vi "process.vi"(1 "input":dbl[][](array[numeric])) -> (0 "xxxx":dbl[][](array[numeric]))   [LabVIEW 2022 SP3]
uses:
  <vilib>/Analysis/NI_AALBase.lvlib
panel:
  out "mean&std":dbl[][](array[numeric])
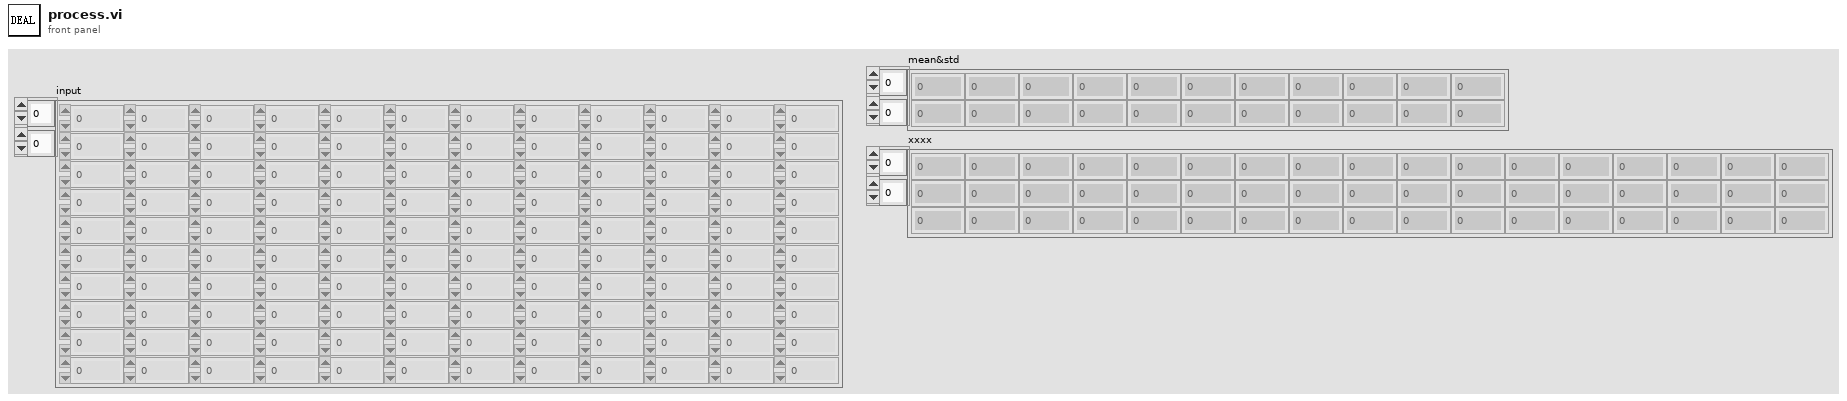
[diagram p1: front panel]
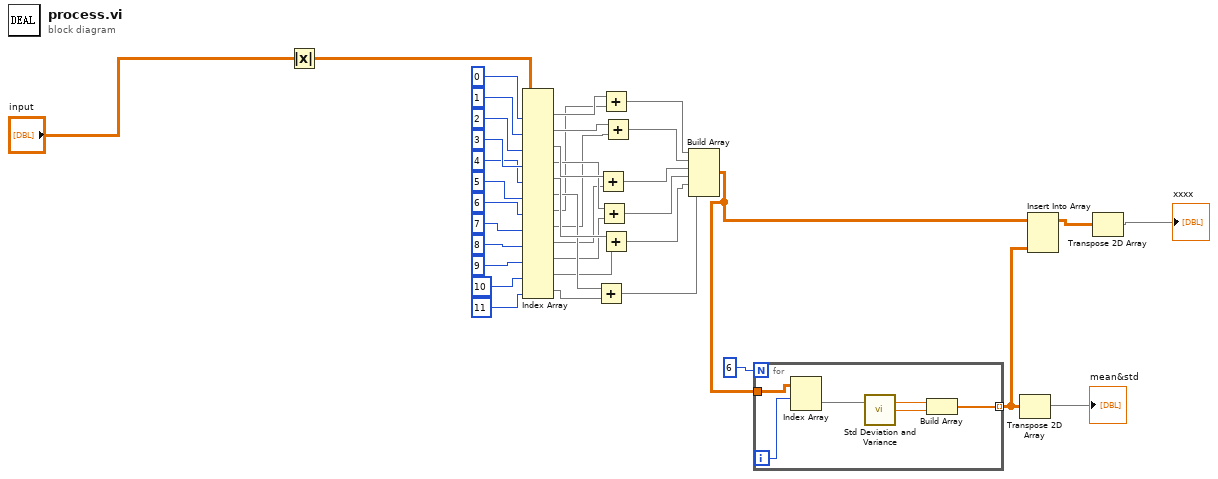
[diagram p0: block diagram]
diagram:
  n1 = Absolute Value(x="input") -> (abs(x)=w2:dbl[][])
  n2 = Index Array(array=w2, index (col) #1=0 ("disabled index (col)"), index (col) #2=1 ("index (col)"), index (col) #3=2 ("index (col)"), index (col) #4=3 ("index (col)"), index (col) #5=4 ("index (col)"), index (col) #6=5 ("index (col)"), index (col) #7=6 ("index (col)"), index (col) #8=7 ("index (col)"), index (col) #9=8 ("index (col)"), index (col) #10=9 ("index (col)"), index (col) #11=10 ("index (col)"), index (col) #12=11 ("index (col)")) -> (element #1=w14:dbl[], element #2=w13:dbl[], element #3=w12:dbl[], element #4=w11:dbl[], element #5=w10:dbl[], element #6=w9:dbl[], element #7=w8:dbl[], element #8=w7:dbl[], element #9=w6:dbl[], element #10=w5:dbl[], element #11=w4:dbl[], element #12=w3:dbl[])  [unwired: 12 in]
  n3 = Add(x=w9, y=w3) -> (x+y=w22:dbl[])
  n4 = Add(x=w12, y=w6) -> (x+y=w1:dbl[])
  n5 = Add(x=w11, y=w5) -> (x+y=w24:dbl[])
  n6 = Add(x=w14, y=w8) -> (x+y=w26:dbl[])
  n7 = Add(x=w10, y=w4) -> (x+y=w23:dbl[])
  n8 = Add(x=w13, y=w7) -> (x+y=w25:dbl[])
  n9 = Build Array(w26, w25, w1, w24, w23, w22) -> (w17:dbl[][])
  n10 = for {
    N: 6 -> [_]
    tunnel: w17 -> [w43]
    tunnel: [w40] -> w16 mode=indexing
    i -> [w39]
    n11 = Index Array(array=w43, index (row)=w39) -> (element=w44:dbl[])  [unwired: 1 in]
    n12 = call <vilib>:"Std Deviation and Variance.vi"("X"=w44) -> ("mean"=w42:dbl, "standard deviation"=w41:dbl)  [unwired: 1 in, 1 out]
    n13 = Build Array(w42, w41) -> (w40:dbl[])
  }
  n14 = Transpose 2D Array(2D array=w16) -> (transposed array=→"mean&std":dbl[][])
  n15 = Insert Into Array(array=w17, new element=w16) -> (w15:dbl[][])  [unwired: 2 in]
  n16 = Transpose 2D Array(2D array=w15) -> (transposed array=→"xxxx":dbl[][])
